vi "Keithley2700-TTTR.vi"(0 "VISA resource name":refnum<visa-resource-name>="COM1", 1 "baud rate":u32=9600, 3 "bytes to read":u32=1000, 4 "data bits":u16=8 min=5 max=8 step=1, 5 "parity":u16(ring) items=["None", "Odd", "Even", "Mark", "Space"], 7 "stop bits":u16(ring)=10 items=["1.0"=10, "1.5"=15, "2.0"=20], 9 "XON Character":u8=17 format="%.0x", 13 "string to write":string="*RST\nFUNC 'TEMP'\nTEMP:TRAN TC\nTEMP:TC:TYPE N\nROUT:CLOS (@101)\nREAD?", 14 "XOFF Character":u8=19 format="%.0x", 15 "timeout (ms)":u32=10000, 17 "write":bool=TRUE, 21 "End read on termination character?":bool=TRUE, 24 "termination char\n(0xA = '\\n' = LF)":u8=10 format="%.0x", 25 "Input\nbuffer size":u32=4096, 26 "read":bool=TRUE) -> (20 "read string":string)   [LabVIEW 2011]
doc: "The Advanced Serial Read and Write example performs a Serial Port Read, a Serial Port Write, or a combination of these actions while setting some advanced serial features like buffer size, termination characters, and XON/XOFF flow control. The user selects the actions (read or write) on the front panel. If both are selected, the VI will write the data first, read the data and then close the VISA session that is opened to the port. \n\nThe parameters set for the serial port must match the parameters of the connected instrument or device. In this example, the bytes to read parameter specifies the number of bytes that the serial port reads. If there were more bytes at the port than the number specified in bytes to read, those bytes would not be read. Also, if you specify to read more bytes than the number of bytes actually read, you might receive a timeout error message.\n\nINSTRUCTIONS:\n1) Select the serial resource and configuration parameters (baud rate, data bits, parity, stop bits, flow control).\n2) Termination character can be enabled and set. Also, set the required input buffer size prior to running the example.\n3) Select the operations to be performed. \n4) Connect the serial port to your device. If no device is available, perform a loopback test by doing one of the following. Short pins 2 and 3 on a RS-232 cable or short pin 4 to pin 8 and pin 5 to pin 9 on a RS-485/422 cable. \n5) Run the VI to see the data read. (The \"read string\" will match the \"string to write\" if a loopback test was performed.)\n\nThis example exposes several advanced features that you may need for your application. Not all applications need all the features shown in this example. The input buffer size is likely an important setting that you want to control in your application. This example expands upon the flow control option for XON and XOFF, allowing the user to choose those control characters. The timeout parameter has been brought to the front panel so a user can specify the time period the VISA Read will wait for the number of bytes to read before timing out. Also, the user has several controls for the termination character, which is discussed later.\n\nNote that you can press the write and read buttons and change the bytes to read parameters on the fly, while the example is running. However, you must stop the example to change the other configuration parameters after the example has started running, and then run again.\n\nSet the I/O buffer size slightly higher the amount of data you expect to receive. This is very important for applications that don't use flow control, as you may lose characters if the receive buffer overflows.\n\nSetting the timeout period ensures that the operation returns with a timeout error if the operation cannot be performed in the specified time period. \n\nSome devices require a termination character in order to identify the end of command strings. Some devices send a termination character to signify the end of data to be read. \n\nThis example shows how you can end the Read operation once a termination character is detected in the buffer and/or append a termination character at the end of the Write data. To enable the Read to end on a termination character, use the VISA Configure Serial Port or use the VISA Properties Serial End Mode for Reads, Termination Character Enable, and Termination Character. To end the Write with a termination character, use the VISA Properties Serial End Mode for Writes, the Send End Enable, and Termination Character. In this example, the same termination character is used for both the Read and the Write. You can specify two different characters for your application, if desired.\n\nYour application may require specific characters for the XON/XOFF Flow Control. You can specify these characters with the VISA Properties Flow Control XOFF Character and Flow Control XON Character. Note that if the standard XON and XOFF characters are used, then decimal 17 and 19 are unavailable for data values. Remember that using flow control and setting an adequate buffer size allow you to prevent buffer overflows."
uses:
  <vilib>/Instr/_visa.llb/VISA Configure Serial Port (Instr).vi
panel:
  out "Waveform Chart":dbl(graph)
  out "Temperatura":dbl
  out "Tiempo":dbl
  out "read string 2":string
  out "actual bytes read":u32
  in  "stop":bool
  in  "flow control":u16(ring) items=["None"=0, "XON/XOFF"=1, "RTS/CTS"=2, "DTR/DSR"=4]
  in  "End write with termination character?":bool=TRUE
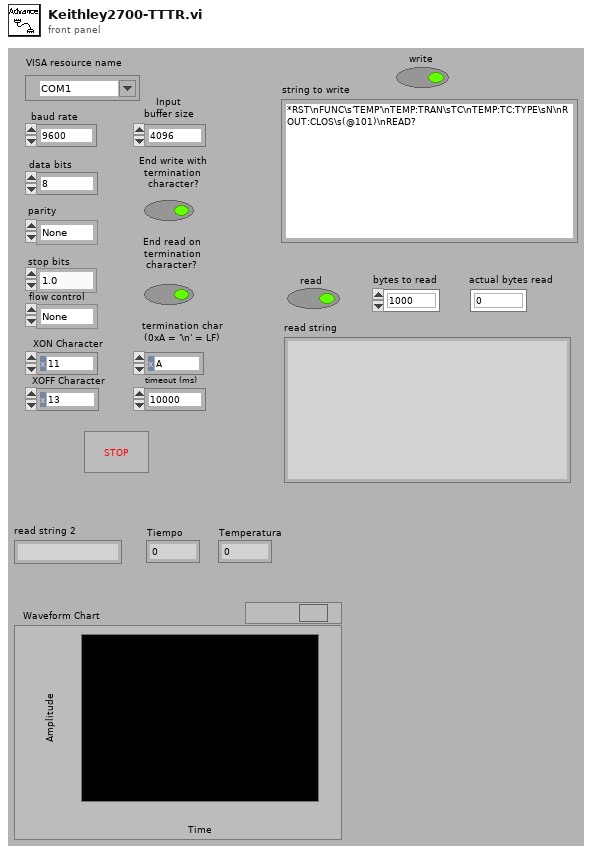
[diagram p1: front panel]
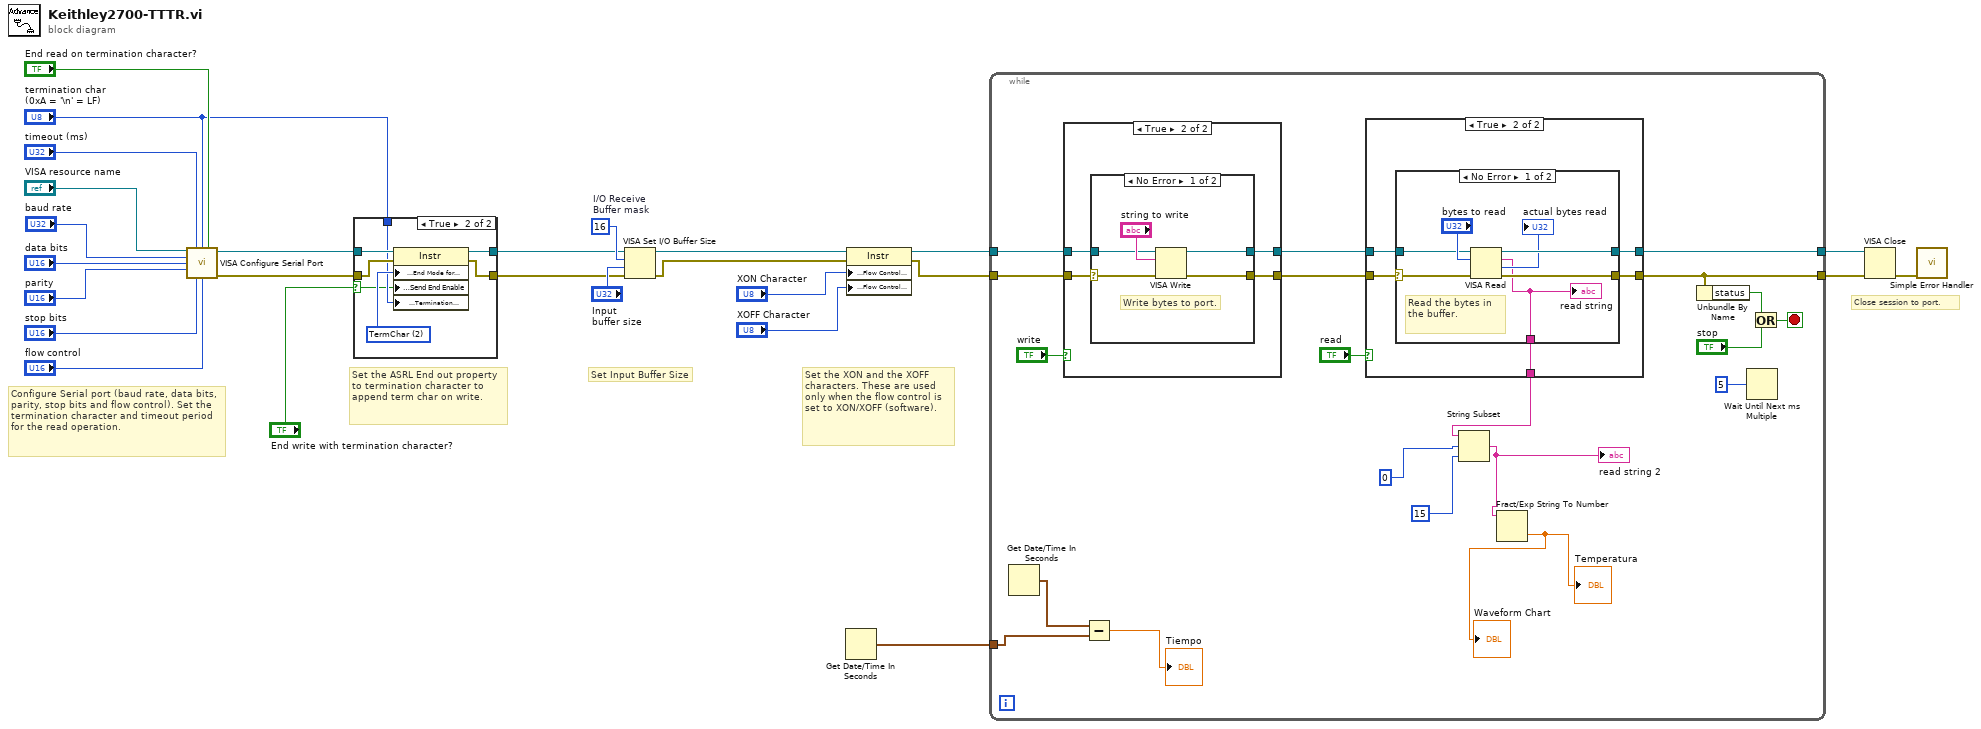
[diagram p0: block diagram]
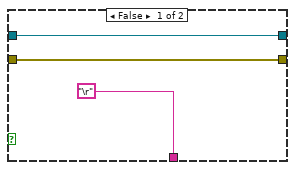
[diagram p5: hidden frame]
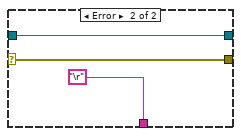
[diagram p6: hidden frame]
diagram:
  w19 = u16 16  # I/O Receive Buffer mask
  # "Set the XON and the XOFF characters. These are used only when the flow control is set to XON/XOFF (software)."
  # "Configure Serial port (baud rate, data bits, parity, stop bits and flow control). Set the termination character and timeout period for the read operation."
  # "Set Input Buffer Size"
  # "Set the ASRL End out property to termination character to append term char on write."
  # "Close session to port."
  n1 = call-poly "VISA Configure Serial Port"("VISA resource name"="VISA resource name", "timeout (10sec)"="timeout (ms)", "termination char\n(0xA = '\\n' = LF)"="termination char\n(0xA = '\\n' = LF)", "Enable Termination\nChar (T)"="End read on termination character?", "baud rate (9600)"="baud rate", "data bits (8)"="data bits", "parity (0:none)"="parity", "stop bits (10: 1 bit)"="stop bits", "flow control (0:none)"="flow control") -> ("VISA resource name out"=w5:refnum<visa-resource-name>, "error out"=w8:errorcluster)  [unwired: 1 in, 4 out]
  n2 = case shown="True" "End write with termination character?" {
    selector: "End write with termination character?" -> [_ w29]
    tunnel: w5 -> [w27 w35]
    tunnel: w8 -> [w28 w34]
    tunnel: [w27 w33] -> w6
    tunnel: [w28 w32] -> w7
    tunnel: "termination char\n(0xA = '\\n' = LF)" -> [_ w30]
    frame False {
    }
    frame True {
      w31 = u16 2 items=["None", "LastBit", "TermChar", "Break"] ("Serial Settings:Serial End Mode for Writes")
      n3 = property on="Property Node" class="Instr"(reference=w35, error in=w34, "Serial Settings:End Mode for Writes"=w31, "Message Based Settings:Send End Enable"=w29, "Message Based Settings:Termination Character"=w30) -> (reference out=w33:refnum<visa-resource-name>, error out=w32:errorcluster)
    }
  }
  n4 = VISA Set I/O Buffer Size(VISA resource name=w6, mask (16)=w19, size (4096)="Input\nbuffer size", error in (no error)=w7) -> (VISA resource name out=w14:refnum<visa-resource-name>, error out=w13:errorcluster)
  n5 = Get Date/Time In Seconds() -> (seconds since 1Jan1904=w1:timestamp)
  n6 = property class="Instr"(reference=w14, error in=w13, "Serial Settings:Flow Control XON Character"="XON Character", "Serial Settings:Flow Control XOFF Character"="XOFF Character") -> (reference out=w4:refnum<visa-resource-name>, error out=w10:errorcluster)
  n7 = while {
    tunnel: w10 -> [w48]
    tunnel: w4 -> [w49]
    tunnel: [w47] -> w3
    tunnel: [w46] -> w2
    tunnel: w1 -> [w39]
    stop <- w45 stop-if-true
    n8 = Get Date/Time In Seconds() -> (seconds since 1Jan1904=w40:timestamp)
    n9 = case shown="True" "write" {
      tunnel: [w57 w61] -> w52
      tunnel: [w56 w60] -> w51
      tunnel: w49 -> [w57 w59]
      tunnel: w48 -> [w56 w58]
      frame False {
      }
      frame True {
        n10 = case shown="No Error" w58 {
          selector: w58 -> [w62 w68]
          tunnel: [w66 w67] -> w61
          tunnel: [w65 w68] -> w60
          tunnel: w59 -> [w63 w67]
          frame No Error {
            # "Write bytes to port."
            n11 = VISA Write(VISA resource name=w63, write buffer="string to write", error in (no error)=w62) -> (VISA resource name out=w66:refnum<visa-resource-name>, error out=w65:errorcluster)  [unwired: 1 out]
          }
          frame Error {
          }
        }
      }
    }
    n12 = Subtract(x=w40, y=w39) -> (x-y=→"Tiempo":dbl)
    n13 = case shown="True" "read" {
      tunnel: w51 -> [w70 w74]
      tunnel: w52 -> [w71 w73]
      tunnel: [w70 w76] -> w46
      tunnel: [w71 w75] -> w47
      tunnel: ["\r" w72] -> w41
      frame False {
      }
      frame True {
        n14 = case "Read bytes from port." shown="No Error" w74 {
          selector: w74 -> [w79 w85]
          tunnel: [w82 w85] -> w76
          tunnel: [w83 w86] -> w75
          tunnel: w73 -> [w80 w86]
          tunnel: [w77 "\r"] -> w72
          frame No Error {
            # "Read the bytes in the buffer."
            n15 = VISA Read(VISA resource name=w80, byte count="bytes to read", error in (no error)=w79) -> (VISA resource name out=w83:refnum<visa-resource-name>, read buffer=w77:string, return count=→"actual bytes read":u32, error out=w82:errorcluster)
            "read string" <- w77
          }
          frame Error {
            # "Error occurred \nreading Bytes at \nSerial Port"
          }
        }
      }
    }
    n16 = String Subset(string=w41, offset (0)=u32 0 ("millisecond multiple"), length (rest)=u32 15 ("millisecond multiple")) -> (substring=w37:string)
    "read string 2" <- w37
    n17 = Fract/Exp String To Number(string=w37) -> (number=→"Temperatura" →"Waveform Chart":dbl)  [unwired: 3 in, 1 out]
    n18 = Unbundle By Name(w46) -> ("status"=w53:bool)
    n19 = Wait Until Next ms Multiple(millisecond multiple=u32 5) -> ()  [unwired: 1 out]
    n20 = Or(x=w53, y="stop") -> (x .or. y?=w45:bool)
  }
  n21 = VISA Close(VISA resource name=w3, error in (no error)=w2) -> (error out=w24:errorcluster)
  n22 = call <vilib>:"Simple Error Handler.vi"("error in (no error)"=w24) -> ()  [unwired: 1 in, 8 out]
